vi "Bertta_v08_1.vi"() -> ()   [LabVIEW 2015]
uses:
  <vilib>/Utility/config.llb/Write Key (I32).vi
  <vilib>/Utility/config.llb/Write Key (String).vi
  <vilib>/Utility/config.llb/Write Key (Double).vi
  <vilib>/Utility/Data Type/NI_Data Type.lvlib
  <vilib>/Utility/config.llb/NI_LVConfig.lvlib
panel:
  out "Started:":string
  in  "SHUTDOWN":bool
  in  "OK Button":bool
  in  "Tab Control":T1(tab)
  in  "Read Seq":bool
  in  "Save Seq":bool
  in  "Configuration file":path=path "C:/Users/shresplab/Desktop/BerttaConfiguration.lvm" caption="Filename"
  in  "OK Button 2":bool
  out "Boolean":bool
  in  "User (initials)":string
  in  "Project name":string
  in  "Description":string
  out "Output file":string
  out "PUMP 1":bool
  out "Target amount":dbl
  out "Scale weight":dbl
  out "Amount now":dbl
  out "Flow rate":dbl
  out "Time to target":dbl format="%<%H:%M:%S>t"
  out "Current step":dbl
  out "Target amount":dbl
  out "Amount now":dbl
  out "Tr":dbl
  out "Tj in":dbl
  out "Tj out":dbl
  out "T set":dbl
  out "Current step":i32
  out "RPM":dbl
  out "Torque 2":dbl
  out "Waveform Chart 5":dynamicdata(graph)
  out "Waveform Chart 6":dynamicdata(graph)
  out "Waveform Chart 7":dynamicdata(graph)
  in  "Tab Control 2":T2(tab)
  out "Waveform Chart 3":dynamicdata(graph)
  out "Waveform Chart 8":dynamicdata(graph)
  out "Waveform Chart 9":dynamicdata(graph)
  out "Table":string[][](table)
  in  "Headers":string[](array[string])=["Flow rate, P1, g/min", "Weight, S1, g", "Amount / step, P1, g", "Step Number, P1", "Total amount, P1, g", "Tj in, C", "Tj out, C", "Tr, C", "RPM", "Torque"]
  in  "T ext / T ext 2":enum32{"T ext", "T ext 2"}(radio)
  out "Sensor OK":bool
  in  "T fail":dbl=20.0
  out "Boolean 12":bool
  out "Boolean 7":bool
  out "Boolean 6":bool
  out "Boolean 5":bool
  out "Boolean 4":bool
  in  "?":bool
  in  "T manual ctrl":dbl=20.0
  in  "Lauda port":dbl=9.0
  out "Data out":dbl
  in  "Bypass select":enum32{"Tr", "Tj"}(radio)
  in  "TempSeq":dbl[][](array[numeric])=[[20.0, 45.0, 50.0, 46.0], [46.0, 50.0, 20.0, 51.0], [20.0, 50.0, 3.0, 25.0], [20.0, 20.0, 0.0, 20.0], [20.0, 20.0, 0.0, 20.0], [20.0, 20.0, 1000.0, 20.0]]
  out "T control":dbl
  out "Tr":dbl
  out "Tj in":dbl
  out "Tj out":dbl
  out "DT":dbl
  out "Elapsed":i32
  in  "PAUSE":bool
  out "Boolean 19":bool
  in  "Reset":bool
  in  "Treshold (Tset)":dbl=1.0
  in  "Tmax":dbl=140.0
  in  "Tmin":dbl=20.0
  out "Current step":i32
  out "Tset":dbl
  out "Waveform Chart":dynamicdata(graph)
  out "External sensor 2":dbl
  out "Data out":dbl
  in  "Port":i32=10
  in  "Radio Buttons":enum32{"Reglo Digital", "Reglo Analog", "PAM"}(radio)
  out "Speed":dbl
  out "mA":dbl format="%#_2g"
  in  "Port":i32=15
  out "RPM":dbl format="%#_2g"
  out "Boolean 18":bool
  out "Boolean 17":bool
  out "Boolean 16":bool
  out "Boolean 15":bool
  out "Boolean 14":bool
  out "Boolean 13":bool
  out "Boolean 11":bool
  out "Boolean 10":bool
  out "Boolean 9":bool
  out "Boolean 8":bool
  in  "PumpSeq":dbl[][](array[numeric])=[[3.0, 3.0, 7.0], [2.0, 2.0, 2.0], [4.0, 2.0, 100.0], [0.0, 0.0, 0.0], [0.0, 0.0, 0.0], [0.0, 0.0, 0.0], [0.0, 0.0, 0.0], [0.0, 0.0, 0.0], [0.0, 0.0, 0.0], [0.0, 0.0, 0.0], [0.0, 1.0, 0.0]]
  in  "?":bool
  out "Flow rate (g/min)":dbl
  out "Time (min)":dbl
  out "Target (g)":dbl
  out "Scale reading":dbl
  out "Step amount now":dbl
  out "Time to target":dbl format="%<%H:%M:%S>t"
  in  "Manual ctrl (g/min)":dbl
  out "Waveform Chart 2":dynamicdata(graph)
  in  "?":bool
  out "Total amount now":dbl
  out "Total time":dbl
  out "Total amount target":dbl
  out "Boolean 20":bool
  in  "Reset 2":bool
  in  "Bypass select 2":enum32{"Remote", "Manual"}(radio)
  in  "Port":dbl=13.0
  out "RPM":dbl
  out "Torque":dbl
  in  "Set RPM":dbl(slide) scale=0.0..500.0
  out "Waveform Chart 4":dynamicdata(graph)
  out "DAQ 9217 (PT100)":errorcluster
  # "PUMP & SCALE 1"
  # "STEP"
  # "TOTAL"
  # "Tinit     >    Tset       min. time       Tfail"
  # "Manual control / end of sequence"
  # "Grams    /   min"
  # "End of sequence"
  # "Pump configuration"
  # "Scale configuration"
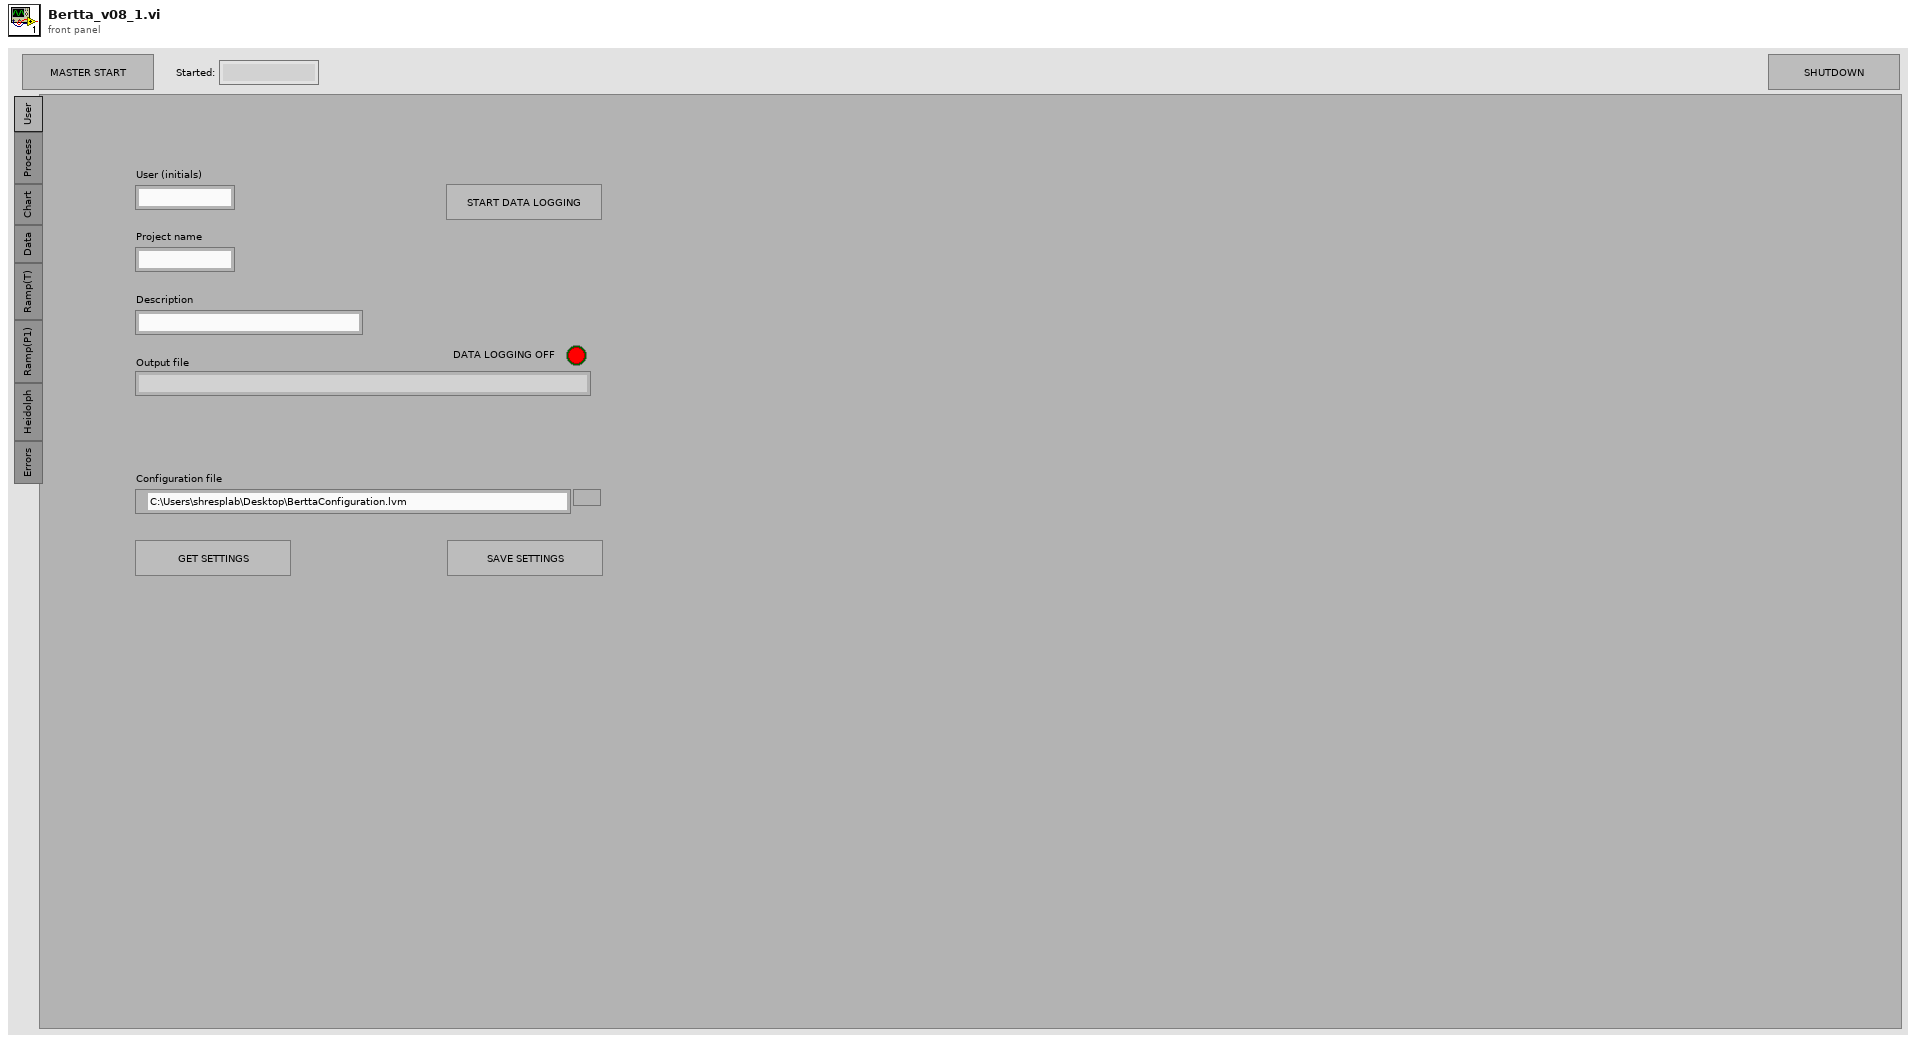
[diagram p1: front panel]
types:
  T1 = enum32{"User", "Process", "Chart", "Data", "Ramp(T)", "Ramp(P1)", "Heidolph", "Errors"}
  T2 = enum32{"Temperatures", "Scale / Pump 1", "RPM / torque"}
  T3 = typedef "NI_LVConfig.lvlib/Config Data RefNum.ctl" = refnum<k1>
  T4 = typedef "NI_Data Type.lvlib/Data Type.ctl" = enum8{"Invalid Type", "Void", "I8", "I16", "I32", "I64", "U8", "U16", "U32", "U64", "Single Float", "Double Float", "Extended Float", "Single Complex", "Double Complex", "Extended Complex", "Enum U8", "Enum U16", "Enum U32", "Enum U64", "Single Float With Unit", "Double Float With Unit", "Extended Float With Unit", "Single Complex with Unit", "Double Complex with Unit", "Extended Complex with Unit", "Boolean", "String", "Path", "Picture", "Tag", "Array", "Cluster", "Variant", "LV Variant", "Waveform", "Timestamp", "Digital Waveform", "Digital Data", "ExpressData", "Refnum", "External Data", "VI", "Poly VI", "LabVIEW Class Instance", "Fixed Point"}
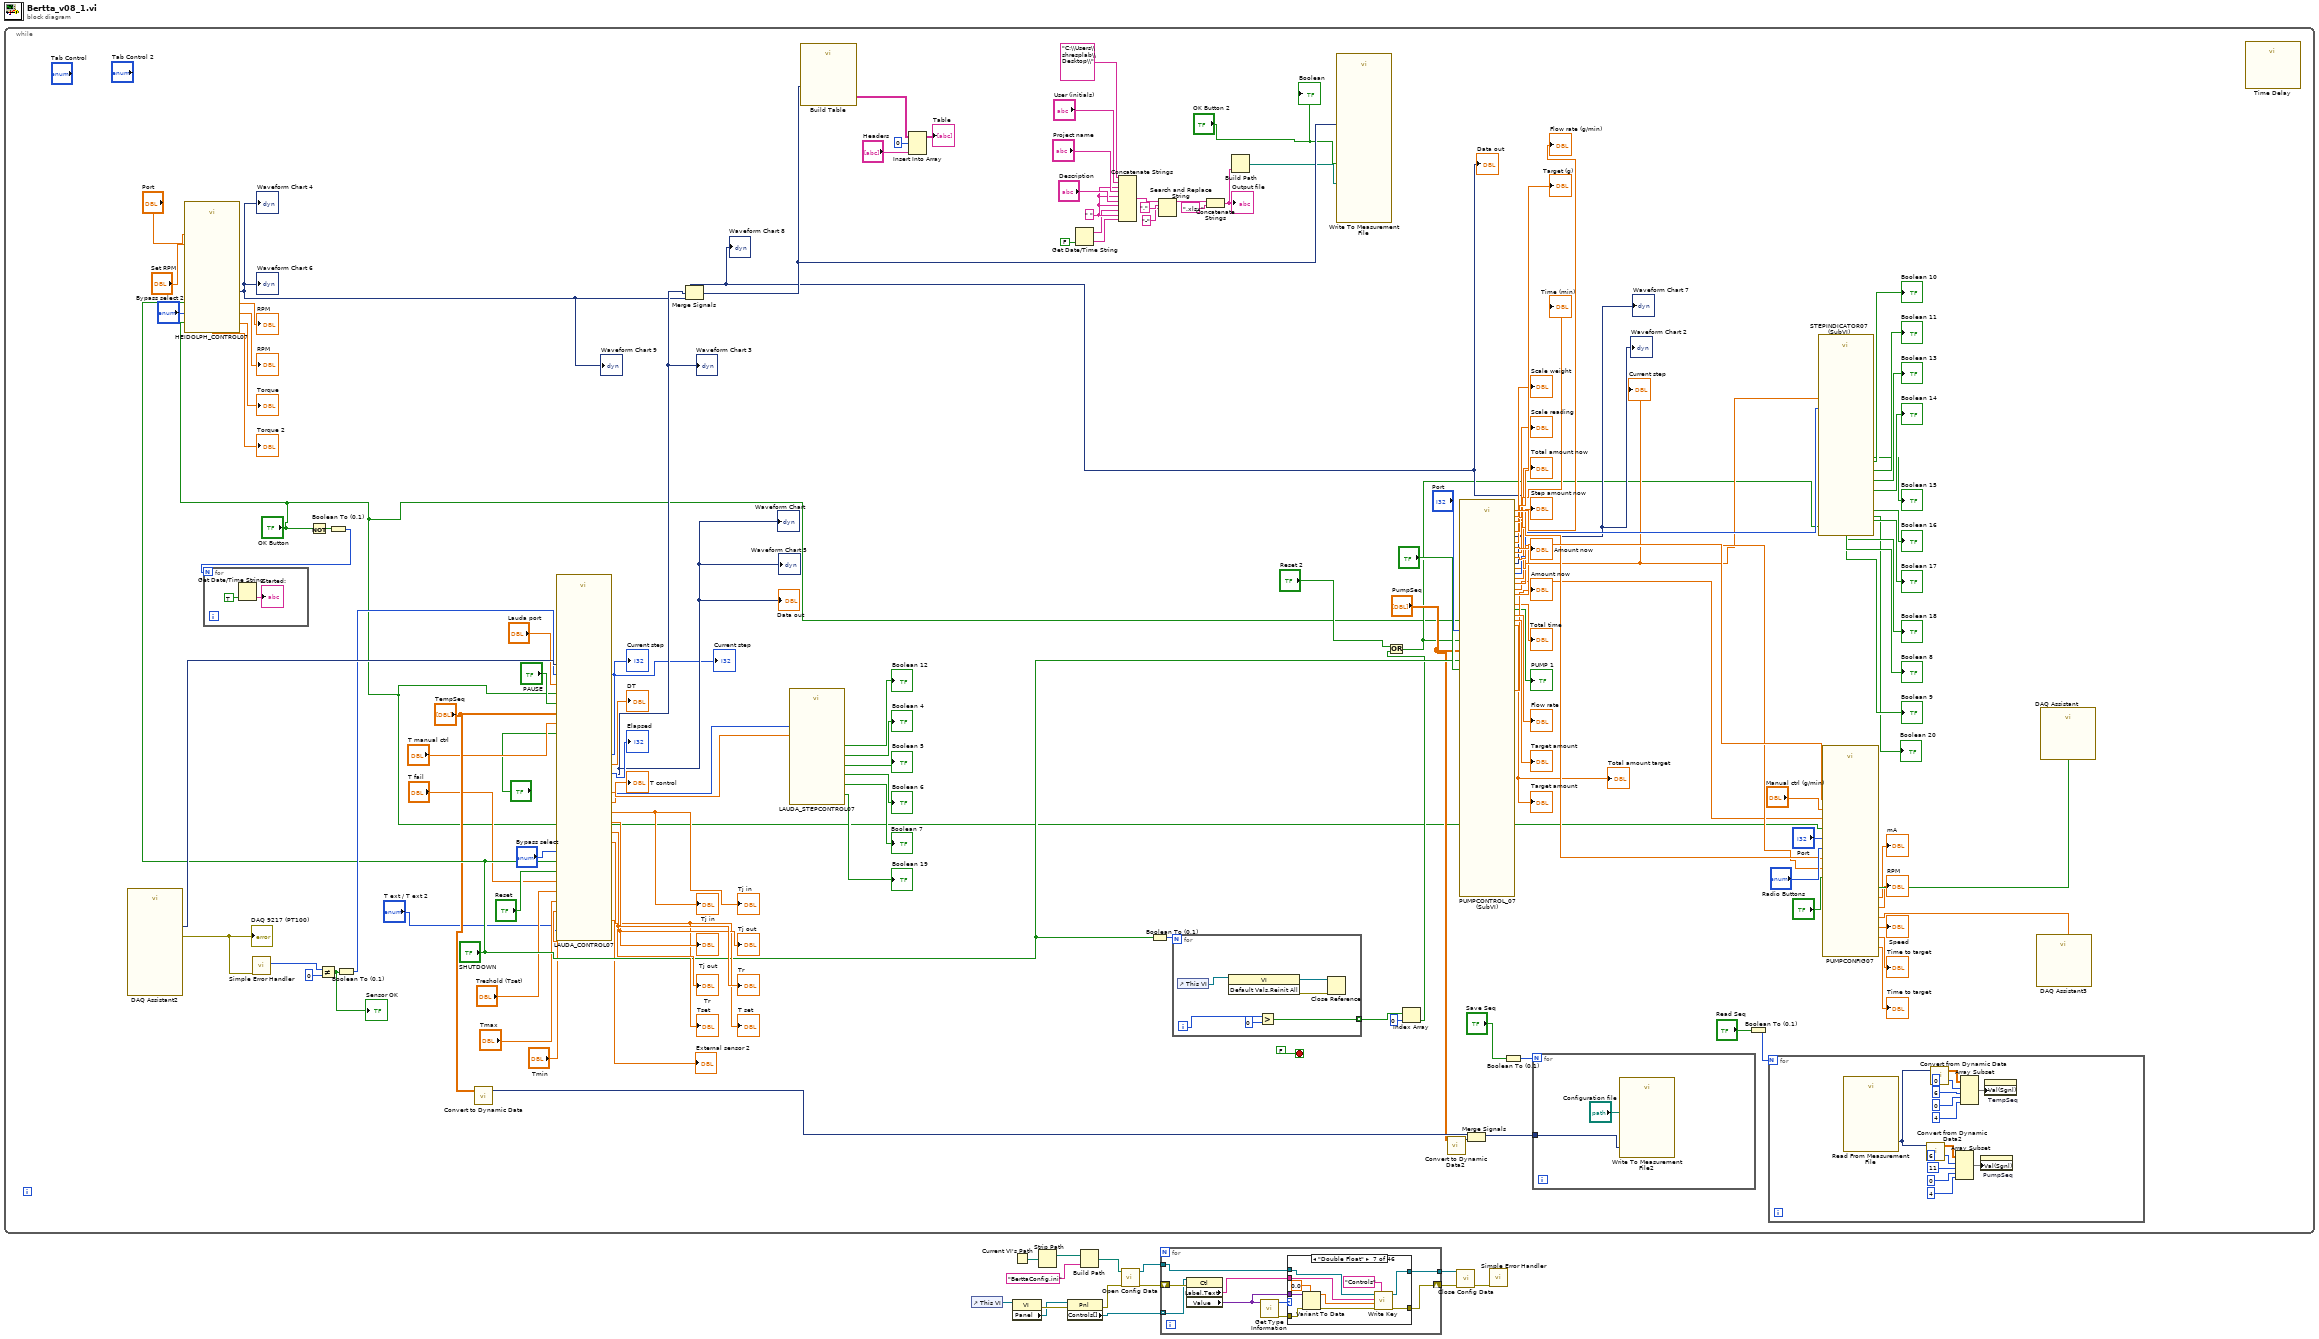
[diagram p0: block diagram]
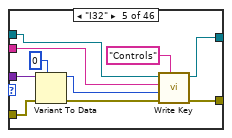
[diagram p6: hidden frame]
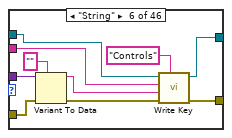
[diagram p7: hidden frame]
diagram:
  n1 = while {
    stop <- FALSE stop-if-true
    w66 = " "
    n2 = call "DAQ Assistant2"() -> ("data"=w133:dynamicdata, "error out"=w74:errorcluster)  [unwired: 17 in, 1 out]
    "DAQ 9217 (PT100)" <- w74
    n3 = call "HEIDOLPH_CONTROL07.vi"("master"="OK Button", "shutdown"="SHUTDOWN", "Bypass select"="Bypass select 2", "Set RPM"="Set RPM", "Device port"="Port") -> ("Dynamic Data"=w80:dynamicdata, "RPM"=→"RPM":dbl, "RPM 2"=→"RPM":dbl, "Torque"=→"Torque":dbl, "Torque 2"=→"Torque 2":dbl)  [unwired: 2 in]
    "Waveform Chart 4" <- w80
    "Waveform Chart 6" <- w80
    "Waveform Chart 9" <- w80
    n4 = call <vilib>:"Simple Error Handler.vi"("error in (no error)"=w74) -> ("code out"=w73:i32)  [unwired: 4 in, 4 out]
    n5 = Not(x="OK Button") -> (.not. x?=w45:bool)
    n6 = Not Equal?(x=w73, y=0) -> (x != y?=w24:bool)
    "Sensor OK" <- w24
    n7 = Boolean To (0,1)(Boolean=w45) -> (0, 1=w46:i16)
    n8 = for {
      N: w46 -> [_]
      n9 = Get Date/Time String(want seconds? (F)=TRUE) -> (time string=→"Started:":string)  [unwired: 2 in, 1 out]
    }
    n10 = Boolean To (0,1)(Boolean=w24) -> (0, 1=w71:i16)
    n11 = call "Convert to Dynamic Data"("2D Array"="TempSeq") -> ("Dynamic Data Type"=w35:dynamicdata)  [unwired: 3 in]
    n12 = call "LAUDA_CONTROL07.vi"("Bypass"="?", "PAUSE"="PAUSE", "data"=w133, "Seq"="TempSeq", "Lauda port"="Lauda port", "Tbypass"="T manual ctrl", "Treshold"="Treshold (Tset)", "Bypass select"="Bypass select", "err"=w71, "Shutdown"="SHUTDOWN", "Master Start"="OK Button", "Reset"="Reset", "Tfail (manual)"="T fail", "Tmax"="Tmax", "T ext / T ext 2"="T ext / T ext 2", "Tmin"="Tmin") -> ("Tj in"=→"Tj in" →"Tj in":dbl, "DT"=→"DT":dbl, "Tj out"=→"Tj out" →"Tj out":dbl, "Tset"=→"Tset" →"T set":dbl, "Dynamic Data"=w82:dynamicdata, "T ext 2"=→"External sensor 2":dbl, "Numeric"=w49:i16, "Numeric 2"=w139:dbl, "T control"=→"T control":dbl, "Current step"=→"Current step" →"Current step":i32, "Elapsed"=→"Elapsed":i32, "Tr"=→"Tr" →"Tr":dbl)
    "Waveform Chart 3" <- w82
    "Waveform Chart" <- w82
    "Data out" <- w82
    "Waveform Chart 5" <- w82
    n13 = call "LAUDA_STEPCONTROL07.vi"("Numeric 2"=w139, "Numeric"=w49) -> ("Boolean 13"=→"Boolean 19":bool, "Boolean 6"=→"Boolean 6":bool, "Boolean 5"=→"Boolean 5":bool, "Boolean 4"=→"Boolean 4":bool, "Boolean 7"=→"Boolean 7":bool, "Boolean 12"=→"Boolean 12":bool)  [unwired: 4 in]
    n14 = Get Date/Time String(want seconds? (F)=FALSE) -> (date string=w65:string, time string=w64:string)  [unwired: 2 in]
    n15 = Concatenate Strings("C:\\Users\\shresplab\\Desktop\\", "User (initials)", w66, "Project name", w66, "Description", w66, w65, w66, w64) -> (w61:string)
    n16 = Boolean To (0,1)(Boolean="SHUTDOWN") -> (0, 1=w42:i16)
    n17 = Search and Replace String(input string=w61, search string=".", replace string="-" ("replace string (\"\")")) -> (result string=w58:string)  [unwired: 5 in, 3 out]
    n18 = for {
      N: w42 -> [_]
      tunnel: [w160] -> w39 mode=indexing
      i -> [w162]
      n19 = control-ref of="This VI"() -> (w165:refnum<vi>)
      n20 = invoke class="VI" method="Default Vals.Reinit All"(reference=w165) -> (reference out=w163:refnum<vi>, error out=w164:errorcluster)  [unwired: 2 in, 1 out]
      n21 = Greater?(x=w162, y=0) -> (0:w160:bool)
      n22 = Close Reference(reference=w163, error in (no error)=w164) -> ()  [unwired: 1 out]
    }
    n23 = Concatenate Strings(w58, ".xlsx") -> (w56:string)
    "Output file" <- w56
    n24 = Build Path(name or relative path=w56) -> (appended path=w70:path)  [unwired: 1 in]
    n25 = Index Array(array=w39, index=0) -> (element=w37:bool)
    n26 = Or(x="Reset 2", y=w37) -> (x .or. y?=w23:bool)
    n27 = call "Convert to Dynamic Data2"("2D Array"="PumpSeq") -> ("Dynamic Data Type"=w33:dynamicdata)  [unwired: 3 in]
    n28 = call "PUMPCONTROL_07 (SubVI).vi"("Port"="Port", "OK Button"="OK Button", 2:"?", "shutdown"="SHUTDOWN", "Seq in"="PumpSeq", "reset"=w23) -> ("Amount now"=→"Amount now":dbl, "Amount now 2"=→"Amount now":dbl, "Flow rate out"=w52:dbl, "Step amount now"=→"Step amount now":dbl, "Total amount now"=→"Total amount now":dbl, "Total time"=→"Total time":dbl, "Numeric 2"=w129:i16, "PUMP 1"=→"PUMP 1":bool, "Numeric"=w125:dbl, "Flow rate"=→"Flow rate":dbl, "Dynamic Data"=w81:dynamicdata, "Target amount"=→"Target amount":dbl, "Time (min) 2"=w130:dbl, "Target amount 2"=→"Total amount target" →"Target amount":dbl, "Scale reading"=→"Scale reading":dbl, "Flow rate (g/min)"=→"Flow rate (g/min)":dbl, "Target (g) 2"=w131:dbl, "Target (g)"=→"Target (g)":dbl, "Time (min)"=→"Time (min)":dbl, "Waveform Chart 2"=→"Waveform Chart 2" →"Waveform Chart 7":dynamicdata, "Scale weight"=→"Scale weight":dbl, "Amount (g)"=w132:dbl)
    "Current step" <- w125
    "Data out" <- w81
    "Waveform Chart 8" <- w81
    n29 = Merge Signals(w81, w82, w80) -> (w83:dynamicdata)
    n30 = call "Build Table"("Signals"=w83) -> ("Table"=w141:string[][])  [unwired: 4 in, 6 out]
    n31 = Insert Into Array(array=w141, index (row)=0, new element="Headers") -> (→"Table":string[][])  [unwired: 1 in]
    n32 = call "Write To Measurement File"("Signals"=w83, "Enable"="OK Button 2", "Filename"=w70) -> ()  [unwired: 14 in, 3 out]
    n33 = Merge Signals(w35, w33) -> (w32:dynamicdata)
    n34 = Boolean To (0,1)(Boolean="Save Seq") -> (0, 1=w31:i16)
    n35 = for {
      N: w31 -> [_]
      tunnel: w32 -> [w159]
      n36 = call "Write To Measurement File2"("Signals"=w159, "Filename"="Configuration file") -> ()  [unwired: 15 in, 3 out]
    }
    n37 = Boolean To (0,1)(Boolean="Read Seq") -> (0, 1=w27:i16)
    n38 = for {
      N: w27 -> [_]
      n39 = call "Read From Measurement File"() -> ("Signals"=w147:dynamicdata)  [unwired: 6 in, 5 out]
      n40 = call "Convert from Dynamic Data2"("Dynamic Data Type"=w147) -> ("Array"=w146:dbl[][])  [unwired: 3 in]
      n41 = call "Convert from Dynamic Data"("Dynamic Data Type"=w147) -> ("Array"=w155:dbl[][])  [unwired: 3 in]
      n42 = Array Subset(array=w146, index (row)=6 ("index"), length (row)=11 ("length"), index (col)=0 ("index"), length (col)=4 ("length")) -> (w145:dbl[][])
      n43 = Array Subset(array=w155, index (row)=0 ("index"), length (row)=6 ("length"), index (col)=0 ("index"), length (col)=4 ("length")) -> (w152:dbl[][])
      n44 = property on="PumpSeq" class="Arr (strict)"("Val(Sgnl)"=w145) -> ()  [unwired: 2 in, 2 out]
      n45 = property on="TempSeq" class="Arr (strict)"("Val(Sgnl)"=w152) -> ()  [unwired: 2 in, 2 out]
    }
    n46 = call "STEPINDICATOR07 (SubVI).vi"("Numeric"=w125, "Numeric 2"=w129, "Reset"=w23) -> ("Boolean 18"=→"Boolean 18":bool, "Boolean 8"=→"Boolean 8":bool, "Boolean 9"=→"Boolean 9":bool, "Boolean 17"=→"Boolean 17":bool, "Boolean 10"=→"Boolean 10":bool, "Boolean 16"=→"Boolean 16":bool, "Boolean 11"=→"Boolean 11":bool, "Boolean 15"=→"Boolean 15":bool, "Boolean 14"=→"Boolean 14":bool, "Boolean 13"=→"Boolean 13":bool, "Boolean 19"=→"Boolean 20":bool)  [unwired: 2 in]
    n47 = call "PUMPCONFIG07.vi"(0:"?", "Radio Buttons"="Radio Buttons", "Bypass (g/min)"="Manual ctrl (g/min)", "Target (g) in"=w131, "Amount (g)"=w132, "Time (min) in"=w130, "Flow rate in"=w52, "OK Button"="OK Button", "Port"="Port") -> ("Time to target 2"=→"Time to target":dbl, "Time to target"=→"Time to target":dbl, "mA"=→"mA":dbl, "signal"=w137:dbl, "Speed"=→"Speed":dbl, "RPM"=→"RPM":dbl, "Array"=w138:bool[])
    n48 = call "DAQ Assistant3"("data"=w137) -> ()  [unwired: 17 in, 2 out]
    n49 = call "DAQ Assistant"("data"=w138) -> ()  [unwired: 17 in, 2 out]
    n50 = call "Time Delay"() -> ()  [unwired: 11 in, 1 out]
    "Boolean" <- "OK Button 2"
  }
  n51 = control-ref of="This VI"() -> (w1:refnum<vi>)
  n52 = property class="VI"(reference=w1) -> (error out=w3:errorcluster, "Panel"=w2:refnum<vi>)  [unwired: 1 in, 1 out]
  n53 = Current VI's Path() -> (path=w5:path)
  n54 = Strip Path(path=w5) -> (stripped path=w6:path)  [unwired: 1 out]
  n55 = property class="Pnl"(reference=w2, error in=w3) -> (error out=w13:errorcluster, "Controls[]"=w4:refnum<vi>[])  [unwired: 1 out]
  n56 = Build Path(base path=w6, name or relative path="BerttaConfig.ini") -> (appended path=w8:path)
  n57 = call <vilib>:"Open Config Data.vi"("error in (no error)"=w13, "configuration file path"=w8) -> ("error out"=w14:errorcluster, "refnum"=w9:T3)  [unwired: 7 in, 1 out]
  n58 = for {
    tunnel: w4 -> [w175] mode=indexing
    tunnel: w9 -> [w171]
    shift-right: [w169] -> w11
    shift-left: w14 -> [w176]
    tunnel: [w170] -> w10
    n59 = property class="Ctl"(reference=w175, error in=w176) -> ("Label.Text"=w172:string, "Value"=w173:variant)  [unwired: 2 out]
    n60 = call <vilib>:"Get Type Information.vi"("Variant"=w173) -> ("error out"=w174:errorcluster, "Type"=w168:T4)  [unwired: 6 in, 3 out]
    n61 = case shown="\"Double Float\"" w168 {
      tunnel: w174 -> [w177 w179 w181 w183 w194 w204 w214 w215 w217 w219 w221 w223 w225 w227 w229 w231 w233 w235 w237 w239 w241 w243 w245 w247 w249 w251 w253 w255 w257 w259 w261 w263 w265 w267 w269 w271 w273 w275 w277 w279 w281 w283 w285 w287 w289 w291]
      tunnel: w173 -> [_ _ _ _ w193 w203 w213 _ _ _ _ _ _ _ _ _ _ _ _ _ _ _ _ _ _ _ _ _ _ _ _ _ _ _ _ _ _ _ _ _ _ _ _ _ _ _]
      tunnel: w172 -> [_ _ _ _ w190 w200 w210 _ _ _ _ _ _ _ _ _ _ _ _ _ _ _ _ _ _ _ _ _ _ _ _ _ _ _ _ _ _ _ _ _ _ _ _ _ _ _]
      tunnel: w171 -> [w178 w180 w182 w184 w189 w199 w209 w216 w218 w220 w222 w224 w226 w228 w230 w232 w234 w236 w238 w240 w242 w244 w246 w248 w250 w252 w254 w256 w258 w260 w262 w264 w266 w268 w270 w272 w274 w276 w278 w280 w282 w284 w286 w288 w290 w292]
      tunnel: [w178 w180 w182 w184 w187 w197 w207 w216 w218 w220 w222 w224 w226 w228 w230 w232 w234 w236 w238 w240 w242 w244 w246 w248 w250 w252 w254 w256 w258 w260 w262 w264 w266 w268 w270 w272 w274 w276 w278 w280 w282 w284 w286 w288 w290 w292] -> w170
      tunnel: [w177 w179 w181 w183 w186 w196 w206 w215 w217 w219 w221 w223 w225 w227 w229 w231 w233 w235 w237 w239 w241 w243 w245 w247 w249 w251 w253 w255 w257 w259 w261 w263 w265 w267 w269 w271 w273 w275 w277 w279 w281 w283 w285 w287 w289 w291] -> w169
      frame "Invalid Type", Default {
      }
      frame "Void" {
      }
      frame "I8" {
      }
      frame "I16" {
      }
      frame "I32" {
        n62 = Variant To Data(error in=w194, type=0, Variant=w193) -> (data=w191:i32, error out=w192:errorcluster)
        n63 = call-poly <vilib>:"Write Key.vi"("section"="Controls", "error in (no error)"=w192, "value"=w191, "key"=w190, "refnum"=w189) -> ("error out"=w186:errorcluster, "refnum out"=w187:T3)  [unwired: 4 in, 1 out]
      }
      frame "String" {
        n64 = Variant To Data(error in=w204, type="", Variant=w203) -> (data=w201:string, error out=w202:errorcluster)
        n65 = call-poly <vilib>:"Write Key.vi"("section"="Controls", "error in (no error)"=w202, "value"=w201, "key"=w200, "refnum"=w199) -> ("error out"=w196:errorcluster, "refnum out"=w197:T3)  [unwired: 4 in, 1 out]
      }
      frame "Double Float" {
        n66 = Variant To Data(error in=w214, type=0.0, Variant=w213) -> (data=w211:dbl, error out=w212:errorcluster)
        n67 = call-poly <vilib>:"Write Key.vi"("section"="Controls", "error in (no error)"=w212, "value"=w211, "key"=w210, "refnum"=w209) -> ("error out"=w206:errorcluster, "refnum out"=w207:T3)  [unwired: 4 in, 1 out]
      }
      frame "I64" {
      }
      frame "U8" {
      }
      frame "U16" {
      }
      frame "U32" {
      }
      frame "U64" {
      }
      frame "Single Float" {
      }
      frame "Extended Float" {
      }
      frame "Single Complex" {
      }
      frame "Double Complex" {
      }
      frame "Extended Complex" {
      }
      frame "Enum U8" {
      }
      frame "Enum U16" {
      }
      frame "Enum U32" {
      }
      frame "Enum U64" {
      }
      frame "Single Float With Unit" {
      }
      frame "Double Float With Unit" {
      }
      frame "Extended Float With Unit" {
      }
      frame "Single Complex with Unit" {
      }
      frame "Double Complex with Unit" {
      }
      frame "Extended Complex with Unit" {
      }
      frame "Boolean" {
      }
      frame "Path" {
      }
      frame "Picture" {
      }
      frame "Tag" {
      }
      frame "Array" {
      }
      frame "Cluster" {
      }
      frame "Variant" {
      }
      frame "LV Variant" {
      }
      frame "Waveform" {
      }
      frame "Timestamp" {
      }
      frame "Digital Waveform" {
      }
      frame "Digital Data" {
      }
      frame "ExpressData" {
      }
      frame "Refnum" {
      }
      frame "External Data" {
      }
      frame "VI" {
      }
      frame "Poly VI" {
      }
      frame "LabVIEW Class Instance" {
      }
      frame "Fixed Point" {
      }
    }
  }
  n68 = call <vilib>:"Close Config Data.vi"("error in (no error)"=w11, "refnum"=w10) -> ("error out"=w12:errorcluster)  [unwired: 8 in, 1 out]
  n69 = call <vilib>:"Simple Error Handler.vi"("error in (no error)"=w12) -> ()  [unwired: 4 in, 5 out]
